vi "SOM.vi"() -> ()   [LabVIEW 2015]
uses:
  SOM_Globals.vi
  <vilib>/httpClient/PUTBuffer.vi
  <vilib>/httpClient/LabVIEWHTTPClient.lvlib
panel:
  out "Current Block":string
  in  "Progress":string
  out "Schedule":string
  in  "Telemetry":T1={"Okay"="OFFLINE", "Robotic"="MANUAL", "Resources"="NONE", "Seeing"=""}
  out "Header Response":string
  out "Body Respponse":string
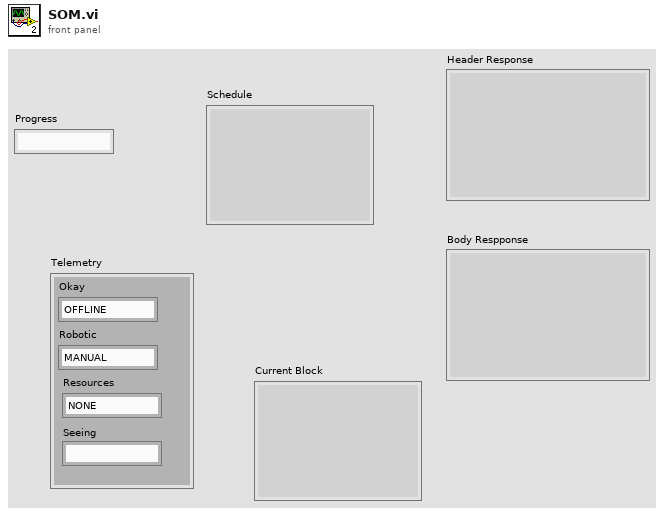
[diagram p1: front panel]
types:
  T1 = cluster{"Okay":string, "Robotic":string, "Resources":string, "Seeing":string}
  T2 = typedef "LabVIEWHTTPClient.lvlib/ClientHandle.ctl" = refnum<k1>
  T3 = cluster{"Mount Az":dbl, "Mount El":dbl, "RA":string, "DEC":string, "Hour Angle":string, "Airmass":dbl, "Focus":dbl, "Rotator Angle":dbl, "Rotator Location":string, "Dome Shutter":string, "Dome Az":dbl, "Date":string, "UT Time":string, "Sidereal Time":string, "Position Angle":dbl, "Seeing":dbl, "OBSRA":string, "OBSDEC":string, "Position ADC":string, "Position ADC 2":string}
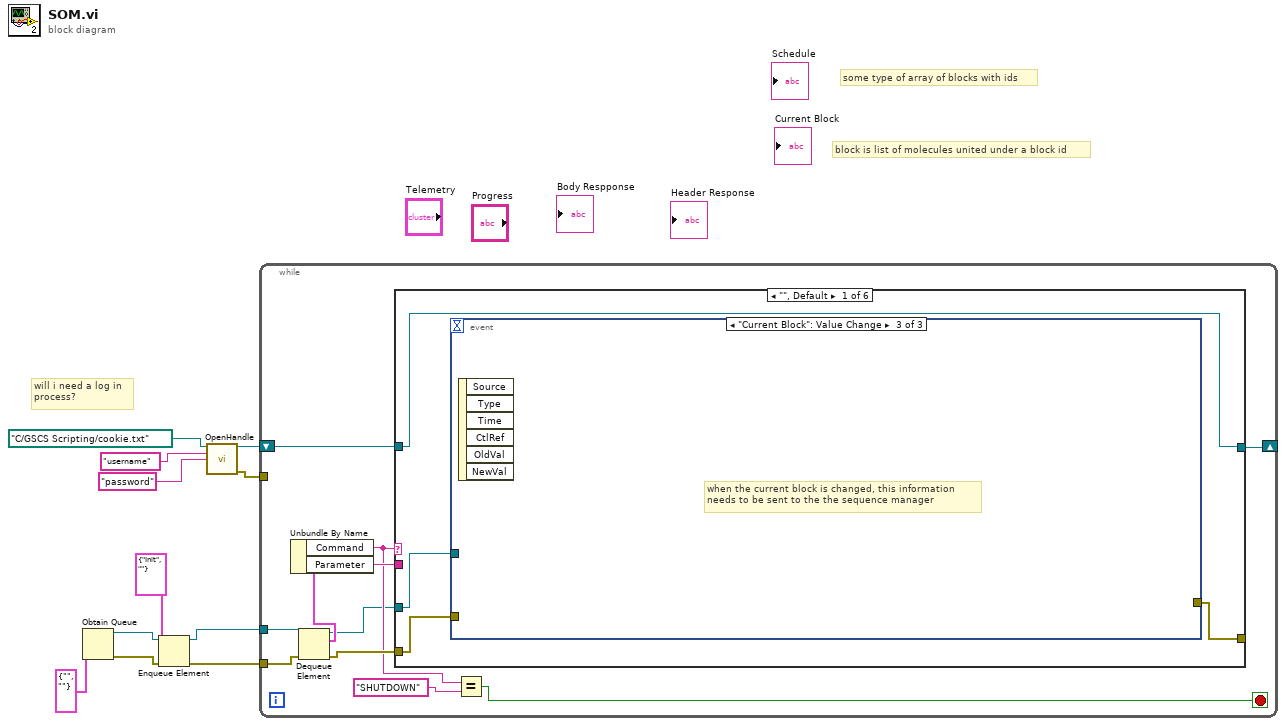
[diagram p0: block diagram]
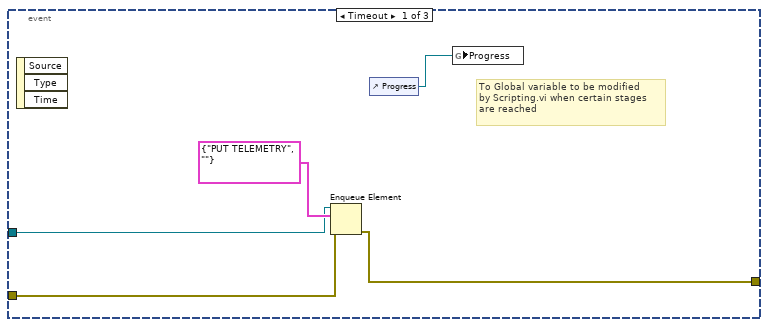
[diagram p2: hidden frame]
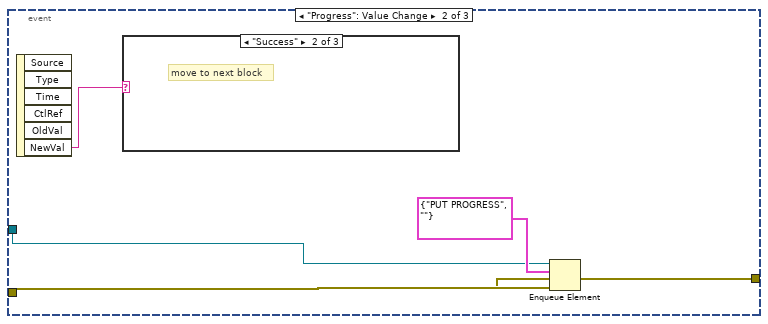
[diagram p3: hidden frame]
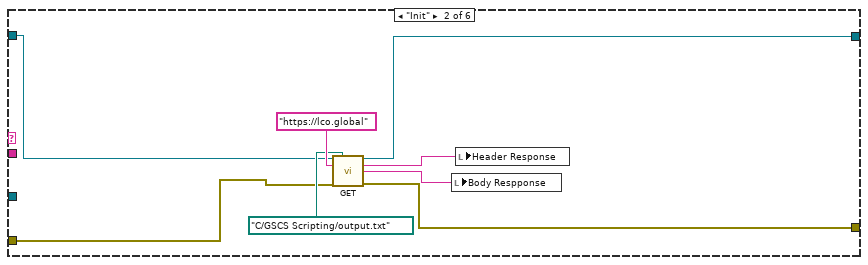
[diagram p6: hidden frame]
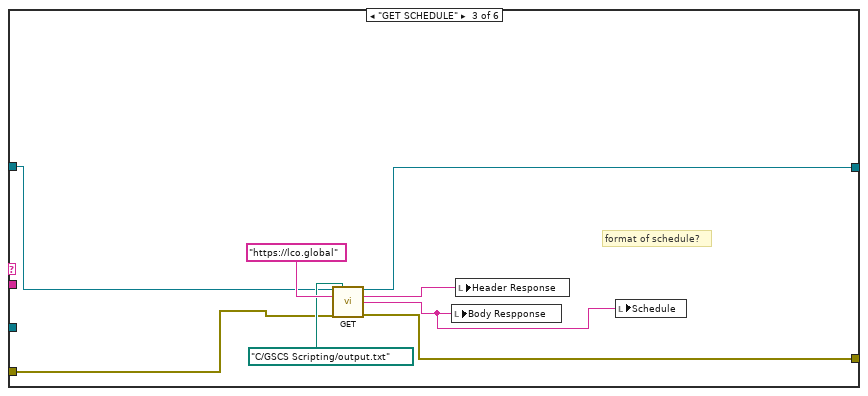
[diagram p7: hidden frame]
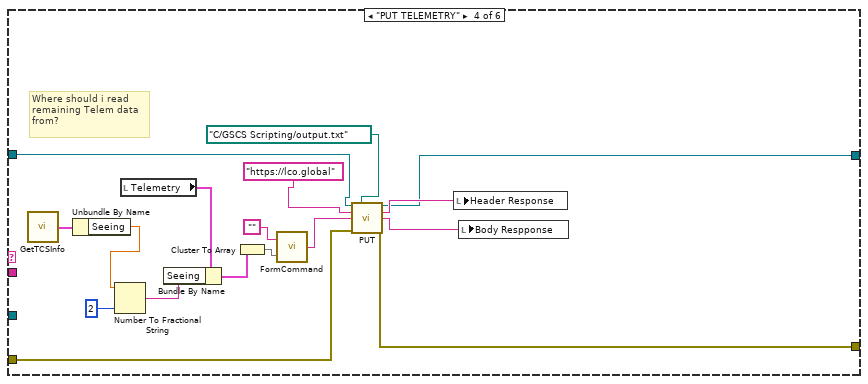
[diagram p8: hidden frame]
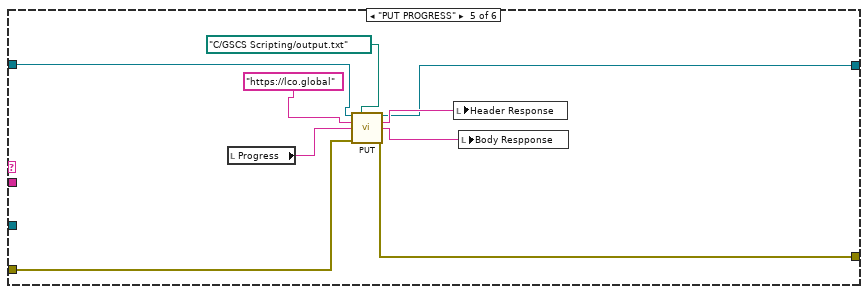
[diagram p9: hidden frame]
diagram:
  # "block is list of molecules united under a block id"
  # "some type of array of blocks with ids"
  # "will i need a log in \nprocess?"
  n1 = Obtain Queue(element data type=cluster{"\nCommand":string, "Parameter":string} {"\nCommand"="", "Parameter"=""}) -> (queue out=w9:refnum<queue>, error out=w8:errorcluster)  [unwired: 4 in, 1 out]
  n2 = Enqueue Element(queue=w9, element=cluster{string, string} {"Init", ""}, error in (no error)=w8) -> (queue out=w7:refnum<queue>, error out=w6:errorcluster)  [unwired: 1 in, 1 out]
  n3 = call <vilib>:"OpenHandle.vi"("cookie file"=path "C:/GSCS Scripting/cookie.txt", "username"="username", "password"="password") -> ("client handle out"=w1:T2, "error out"=w2:errorcluster)  [unwired: 11 in]
  n4 = while {
    tunnel: w7 -> [w22]
    tunnel: w6 -> [w21]
    tunnel: w2 -> [_]
    shift-right: [w12] -> _
    shift-left: w1 -> [w17]
    stop <- w14 stop-if-true
    n5 = Dequeue Element(queue=w22, error in (no error)=w21) -> (queue out=w13:refnum<queue>, element=w20:cluster{"\nCommand":string, "Parameter":string}, error out=w18:errorcluster)  [unwired: 1 in, 1 out]
    n6 = Unbundle By Name(w20) -> ("Command"=w15:string, "Parameter"=w19:string)
    n7 = case shown="\"\", Default" w15 {
      tunnel: w19 -> [_ _ _ _ _ _]
      tunnel: w18 -> [w25 w40 w49 w58 w72 w79]
      tunnel: w17 -> [w24 w39 w48 w67 w76 w80]
      tunnel: w13 -> [w26 _ _ _ _ _]
      tunnel: [w24 w38 w47 w59 w73 w80] -> w12
      tunnel: [w23 w37 w46 w57 w71 w79] -> _
      frame "", Default {
        n8 = event shown="[2] \"Current Block\": Value Change" {
          selector: _ -> [_ _ _]
          dyn-events: _ -> [_ _ _]
          timeout: _ -> [_ _ _]
          tunnel: w26 -> [w30 w35 _]
          tunnel: w25 -> [w29 w34 _]
          tunnel: [w28 w33 _] -> w23
          event Timeout {
            # "To Global variable to be modified\nby Scripting.vi when certain stages \nare reached"
            n9 = event-data() -> ()  [unwired: 1 in, 3 out]
            n10 = Enqueue Element(queue=w30, element=cluster{string, string} {"PUT TELEMETRY", ""}, error in (no error)=w29) -> (error out=w28:errorcluster)  [unwired: 1 in, 2 out]
            n11 = control-ref of="Progress"() -> (w27:refnum<vi>)
            n12 = global write "SOM_Globals.vi" "Progress"(w27) -> ()
          }
          event "Progress": Value Change {
            n13 = event-data() -> ("NewVal"=w32:string)  [unwired: 1 in, 5 out]
            n14 = case shown="\"Success\"" w32 {
              frame "Fail", Default {
                # "get report"
              }
              frame "Success" {
                # "move to next block"
              }
              frame "Attempted" {
                # "Nothing needs to happen here"
              }
            }
            n15 = Enqueue Element(queue=w35, element=cluster{string, string} {"PUT PROGRESS", ""}, error in (no error)=w34) -> (error out=w33:errorcluster)  [unwired: 1 in, 2 out]
          }
          event "Current Block": Value Change {
            # "when the current block is changed, this information\nneeds to be sent to the the sequence manager"
            n16 = event-data() -> ()  [unwired: 1 in, 6 out]
          }
        }
      }
      frame "Init" {
        n17 = call <vilib>:"GET.vi"("client handle"=w39, "output file"=path "C:/GSCS Scripting/output.txt", "url"="https://lco.global", "error in (no error)"=w40) -> ("client handle out"=w38:T2, "headers"=w42:string, "body"=w41:string, "error out"=w37:errorcluster)  [unwired: 8 in]
        n18 = local write "Body Respponse"(w41) -> ()
        n19 = local write "Header Response"(w42) -> ()
      }
      frame "GET SCHEDULE" {
        # "format of schedule?"
        n20 = call <vilib>:"GET.vi"("client handle"=w48, "output file"=path "C:/GSCS Scripting/output.txt", "url"="https://lco.global", "error in (no error)"=w49) -> ("client handle out"=w47:T2, "headers"=w50:string, "body"=w45:string, "error out"=w46:errorcluster)  [unwired: 8 in]
        n21 = local write "Body Respponse"(w45) -> ()
        n22 = local write "Header Response"(w50) -> ()
        n23 = local write "Schedule"(w45) -> ()
      }
      frame "PUT TELEMETRY" {
        # "Where should i read \nremaining Telem data\nfrom?"
        n24 = call "GetTCSInfo.vi"() -> ("TCSInfo"=w66:T3)
        n25 = Unbundle By Name(w66) -> ("Seeing"=w64:dbl)
        n26 = Number To Fractional String(number=w64, precision (6)=2) -> (F-format string=w63:string)  [unwired: 2 in]
        n27 = local read "Telemetry"() -> (w65:T1)
        n28 = Bundle By Name(cluster=w65, "Seeing"=w63) -> (w55:T1)
        n29 = Cluster To Array(cluster=w55) -> (array=w54:string[])
        n30 = call "FormCommand.vi"("Parameters"=w54, "Command"="") -> ("Command string"=w56:string)
        n31 = call-poly <vilib>:"PUT.vi"("client handle"=w67, "output file"=path "C:/GSCS Scripting/output.txt", "url"="https://lco.global", "buffer"=w56, "error in (no error)"=w58) -> ("client handle out"=w59:T2, "headers"=w61:string, "body"=w60:string, "error out"=w57:errorcluster)  [unwired: 7 in]
        n32 = local write "Header Response"(w61) -> ()
        n33 = local write "Body Respponse"(w60) -> ()
      }
      frame "PUT PROGRESS" {
        n34 = local read "Progress"() -> (w70:string)
        n35 = call-poly <vilib>:"PUT.vi"("client handle"=w76, "output file"=path "C:/GSCS Scripting/output.txt", "url"="https://lco.global", "buffer"=w70, "error in (no error)"=w72) -> ("client handle out"=w73:T2, "headers"=w75:string, "body"=w74:string, "error out"=w71:errorcluster)  [unwired: 7 in]
        n36 = local write "Header Response"(w75) -> ()
        n37 = local write "Body Respponse"(w74) -> ()
      }
      frame "Send Block" {
        # "send block over to sequence manager, if accepted - attempted"
      }
    }
    n38 = Equal?(x=w15, y="SHUTDOWN") -> (x = y?=w14:bool)
  }
